vi "InitSensor.vi"   [LabVIEW 2018]
uses:
  <vilib>/Rock Robotics/SystemInterfaces/AI/FPGA_AIChannel.ctl
  refnums.vi
types:
  T1 = typedef "FPGA_AIChannel.ctl" = enum8{"AI 0", "AI 1", "AI 2", "AI 3", "AI MXP 0", "AI MXP 1", "AI MXP 2", "AI MXP 3", "Invalid"}
  T2 = typedef "WPI_PotentiometerDevRef.ctl" = cluster{"DevStatus":errorcluster, "Analog Channel":T1, "Invert Output":bool}
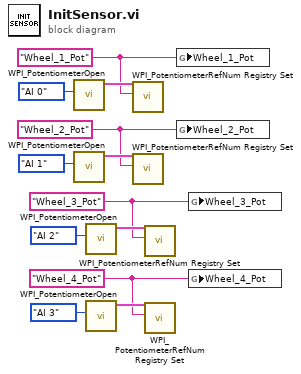
[diagram p0: block diagram]
diagram:
  w1 = "Wheel_4_Pot"
  w4 = "Wheel_3_Pot"
  w7 = "Wheel_2_Pot"
  w10 = "Wheel_1_Pot"
  n1 = call <vilib>:"WPI_PotentiometerOpen.vi"("Analog Channel"=FPGA_AIChannel."AI 0") -> ("PotDevRef"=w12:T2)  [unwired: 9 in, 1 out]
  n2 = call <vilib>:"WPI_PotentiometerOpen.vi"("Analog Channel"=FPGA_AIChannel."AI 1") -> ("PotDevRef"=w9:T2)  [unwired: 9 in, 1 out]
  n3 = call <vilib>:"WPI_PotentiometerOpen.vi"("Analog Channel"=FPGA_AIChannel."AI 2") -> ("PotDevRef"=w6:T2)  [unwired: 9 in, 1 out]
  n4 = call <vilib>:"WPI_PotentiometerOpen.vi"("Analog Channel"=FPGA_AIChannel."AI 3") -> ("PotDevRef"=w3:T2)  [unwired: 9 in, 1 out]
  n5 = call <vilib>:"WPI_PotentiometerRefNum Registry Set.vi"("refnum name"=w10, "PotDevRef"=w12) -> ()  [unwired: 8 in, 2 out]
  n6 = call <vilib>:"WPI_PotentiometerRefNum Registry Set.vi"("refnum name"=w7, "PotDevRef"=w9) -> ()  [unwired: 8 in, 2 out]
  n7 = call <vilib>:"WPI_PotentiometerRefNum Registry Set.vi"("refnum name"=w4, "PotDevRef"=w6) -> ()  [unwired: 8 in, 2 out]
  n8 = call <vilib>:"WPI_PotentiometerRefNum Registry Set.vi"("refnum name"=w1, "PotDevRef"=w3) -> ()  [unwired: 8 in, 2 out]
  n9 = global write "refnums.vi" "Wheel_1_Pot"(w10) -> ()
  n10 = global write "refnums.vi" "Wheel_2_Pot"(w7) -> ()
  n11 = global write "refnums.vi" "Wheel_3_Pot"(w4) -> ()
  n12 = global write "refnums.vi" "Wheel_4_Pot"(w1) -> ()
